vi "Client TCP Request Version.vi"(8 "error in (no error)":errorcluster, 11 "Client IP":string) -> (0 "error out":errorcluster, 1 "Client Version":T1 {"Build Date/Time" format="%<%X\n%x>T"}, 2 "Client Detected?":bool, 3 "Client Version String":string)   [LabVIEW 2011]
uses:
  SI.LIB/OGAB Version.ctl
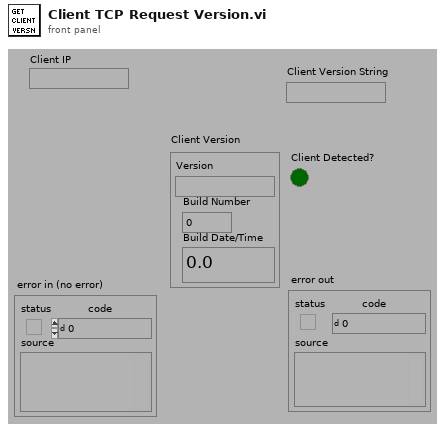
[diagram p1: front panel]
types:
  T1 = typedef "OGAB Version.ctl" = cluster{"Version":string, "Build Number":u32, "Build Date/Time":dbl}
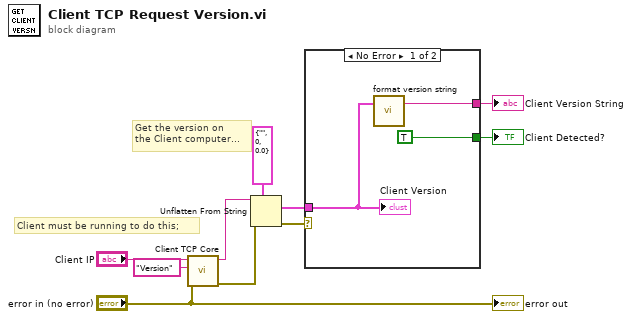
[diagram p0: block diagram]
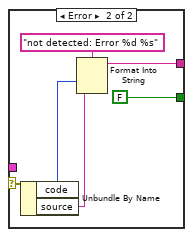
[diagram p2: hidden frame]
diagram:
  # "Client must be running to do this;"
  # "Get the version on \nthe Client computer..."
  n1 = call "Client TCP Core.vi"("error in (no error)"="error in (no error)", "Command(Params) (\"\")"="Version" ("Command(Params) (\"\")"), "Client (\"\": localhost)"="Client IP") -> ("error out"=w2:errorcluster, "ACKed Response"=w8:string)  [unwired: 7 out]
  n2 = Unflatten From String(type=T1 {"Version"="", "Build Number"=0, "Build Date/Time"=0.0} ("Version"), binary string=w8, error in (no error)=w2) -> (value=w6:T1, error out=w3:errorcluster)  [unwired: 3 out]
  n3 = case shown="No Error" w3 {
    selector: w3 -> [_ w18]
    tunnel: [w12 w16] -> w9
    tunnel: [TRUE FALSE] -> w10
    tunnel: w6 -> [w11 _]
    frame No Error {
      n4 = call "format version string.vi"("Version"=w11) -> ("Version String"=w12:string)  [unwired: 2 out]
      "Client Version" <- w11
    }
    frame Error {
      n5 = Unbundle By Name(w18) -> ("code"=w15:i32, "source"=w14:string)
      n6 = Format Into String(format string="not detected: Error %d %s" ("Template (\"\")"), w15, w14) -> (resulting string=w16:string)  [unwired: 2 in, 1 out]
    }
  }
  "Client Detected?" <- w10
  "Client Version String" <- w9
  "error out" <- "error in (no error)"
